vi "PLC_Control_Init.vi"(2 "Mode":enum16{"RTU", "ASCII"}(ring), 3 "Flow Control":u16(ring) items=["None", "XON/XOFF", "RTS/CTS", "XON/XOFF & RTS/CTS", "DTR/DSR", "XON/XOFF & DTR/DSR"], 4 "error in (no error)":errorcluster, 5 "Baud Rate":u32=9600, 6 "Parity":u16(ring) items=["None", "Odd", "Even", "Mark", "Space"], 7 "VISA resource name":refnum<visa-resource-name>) -> (0 "error out":errorcluster, 1 "VISA resource name out":refnum<visa-resource-name>)   [LabVIEW 2015]
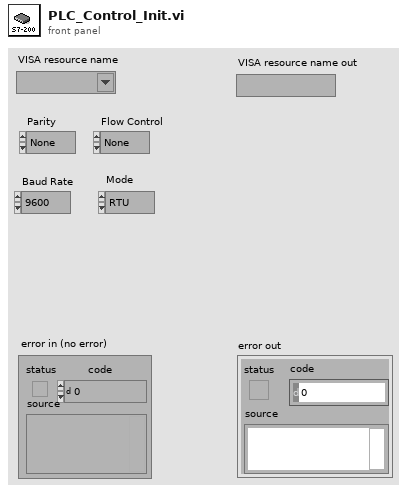
[diagram p1: front panel]
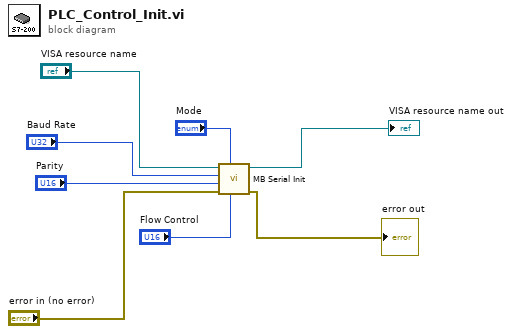
[diagram p0: block diagram]
diagram:
  n1 = call "MB Serial Init.vi"("Flow Control"="Flow Control", "Mode"="Mode", "error in (no error)"="error in (no error)", "Parity"="Parity", "Baud Rate"="Baud Rate", "VISA resource name"="VISA resource name") -> ("error out"=→"error out":errorcluster, "VISA resource name out"=→"VISA resource name out":refnum<visa-resource-name>)  [unwired: 4 in]
